vi "Control Panel Controller.vi"(8 "error in":errorcluster) -> ()   [LabVIEW 2019]
doc: "This VI executes continuously carrying out the current operation and responding to updates or new operations. It will often contain the timing or control code that is difficult to place directly in TeleOp. This VI generally opens all sensors and motors and isolates the rest of the robot code from knowing how the operations are carried out."
uses:
  <vilib>/Rock Robotics/WPI/Framework/Completion Status.ctl
  Control Panel Setpoints.ctl
  Control Panel Operations.ctl
  <vilib>/Rock Robotics/WPI/ThirdParty/Phoenix-LabVIEW/Motor Controller/Controls/CTRE_Phoenix_MotorControl_ControlMode.ctl
  Framework/Robot Global Data.vi
  <vilib>/Rock Robotics/Network Tables/NT Write Number.vi
panel:
  in  "Interactive Values":T1
  out "Current\nCmd":string
  in  "Buttons":cluster{"Execute Cmd":bool, "Abort Cmd":bool}
  out "Command Timing":cluster{"Start Time (ms)":u32, "Iterations":i32}
  out "Status":T3
  # "Tip: It may be helpful to observe inputs and sensor values.\nYou may also want to display tuning or debugging controls."
  # "Interactive Command: You may fill in the settings for a command\nand schedule it with the Execute button. You can observe and abort\nany command while fine tuning the code for the controller."
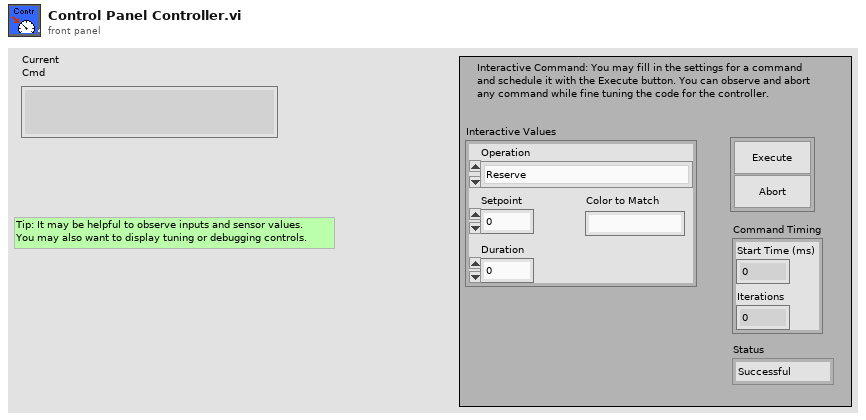
[diagram p1: front panel]
types:
  T1 = typedef "Control Panel Setpoints.ctl" = cluster{"Operation":T2, "Setpoint":dbl, "Duration":dbl, "Color to Match":string}
  T2 = typedef "Control Panel Operations.ctl" = enum16{"Reserve", "Read Current", "Immediate", "Move for Time", "Three Turns", "Match Color"}
  T3 = typedef "Completion Status.ctl" = enum16{"Successful", "Aborted", "Incomplete"}
  T4 = typedef "WPI_MotorControlDeviceRef.ctl" = cluster{"DeviceStatus":errorcluster, "Type":T5, "PWM":cluster{"PWM Channel":T6, "DeadBand":T7}, "CAN":cluster{"Device Number":u8, "SetOutput VI Ref":variant, "GetOutput VI Ref":variant, "Enable VI Ref":variant, "Disable VI Ref":variant, "Data":variant}, "Invert":bool, "DIO PWM":cluster{"PWM \"Enable\" Channel":T6, "DIOChannel":T8, "PWM Rate":dbl}}
  T5 = typedef "WPI_MotorControlType.ctl" = enum16{"PWM", "CAN", "DIO PWM"}
  T6 = typedef "FPGA_DIOPWMChannel.ctl" = enum8{"PWM 0", "PWM 1", "PWM 2", "PWM 3", "PWM 4", "PWM 5", "PWM 6", "PWM 7", "PWM 8", "PWM 9", "PWM MXP 0", "PWM MXP 1", "PWM MXP 2", "PWM MXP 3", "PWM MXP 4", "PWM MXP 5", "PWM MXP 6", "PWM MXP 7", "PWM MXP 8", "PWM MXP 9", "Invalid"}
  T7 = typedef "WPI_PWMDeadband.ctl" = cluster{"Name":string, "maxPositivePwm":i32, "minPositivePwm":i32, "centerPwm":i32, "maxNegativePwm":i32, "minNegativePwm":i32, "angularRange":u16}
  T8 = typedef "FPGA_DIOChannel.ctl" = enum8{"DIO 0", "DIO 1", "DIO 2", "DIO 3", "DIO 4", "DIO 5", "DIO 6", "DIO 7", "DIO 8", "DIO 9", "DIO MXP 0", "DIO MXP 1", "DIO MXP 2", "DIO MXP 3", "DIO MXP 4", "DIO MXP 5", "DIO MXP 6", "DIO MXP 7", "DIO MXP 8", "DIO MXP 9", "DIO MXP 10", "DIO MXP 11", "DIO MXP 12", "DIO MXP 13", "DIO MXP 14", "DIO MXP 15", "SPI Port CS1", "SPI Port CS2", "SPI Port CS3", "SPI Port MISO", "SPI Port MOSI", "Invalid"}
  T9 = typedef "Command Status Info.ctl" = cluster{"Name":string, "Status":T3, "notifier out":T10}
  T10 = typedef "Completion Notifier.ctl" = refnum<notifier>
  T11 = cluster{"Current Command":T1, "Command Timing":cluster{"Start Time (ms)":u32, "Iterations":i32}, "Command Arguments":cluster{"Command Info":T9, "Description":string, "Default Command":T1, "queue out":refnum<queue>, "Subsystem Name":string}}
  T12 = typedef "CTRE_Phoenix_MotorControl_ControlMode.ctl" = u16
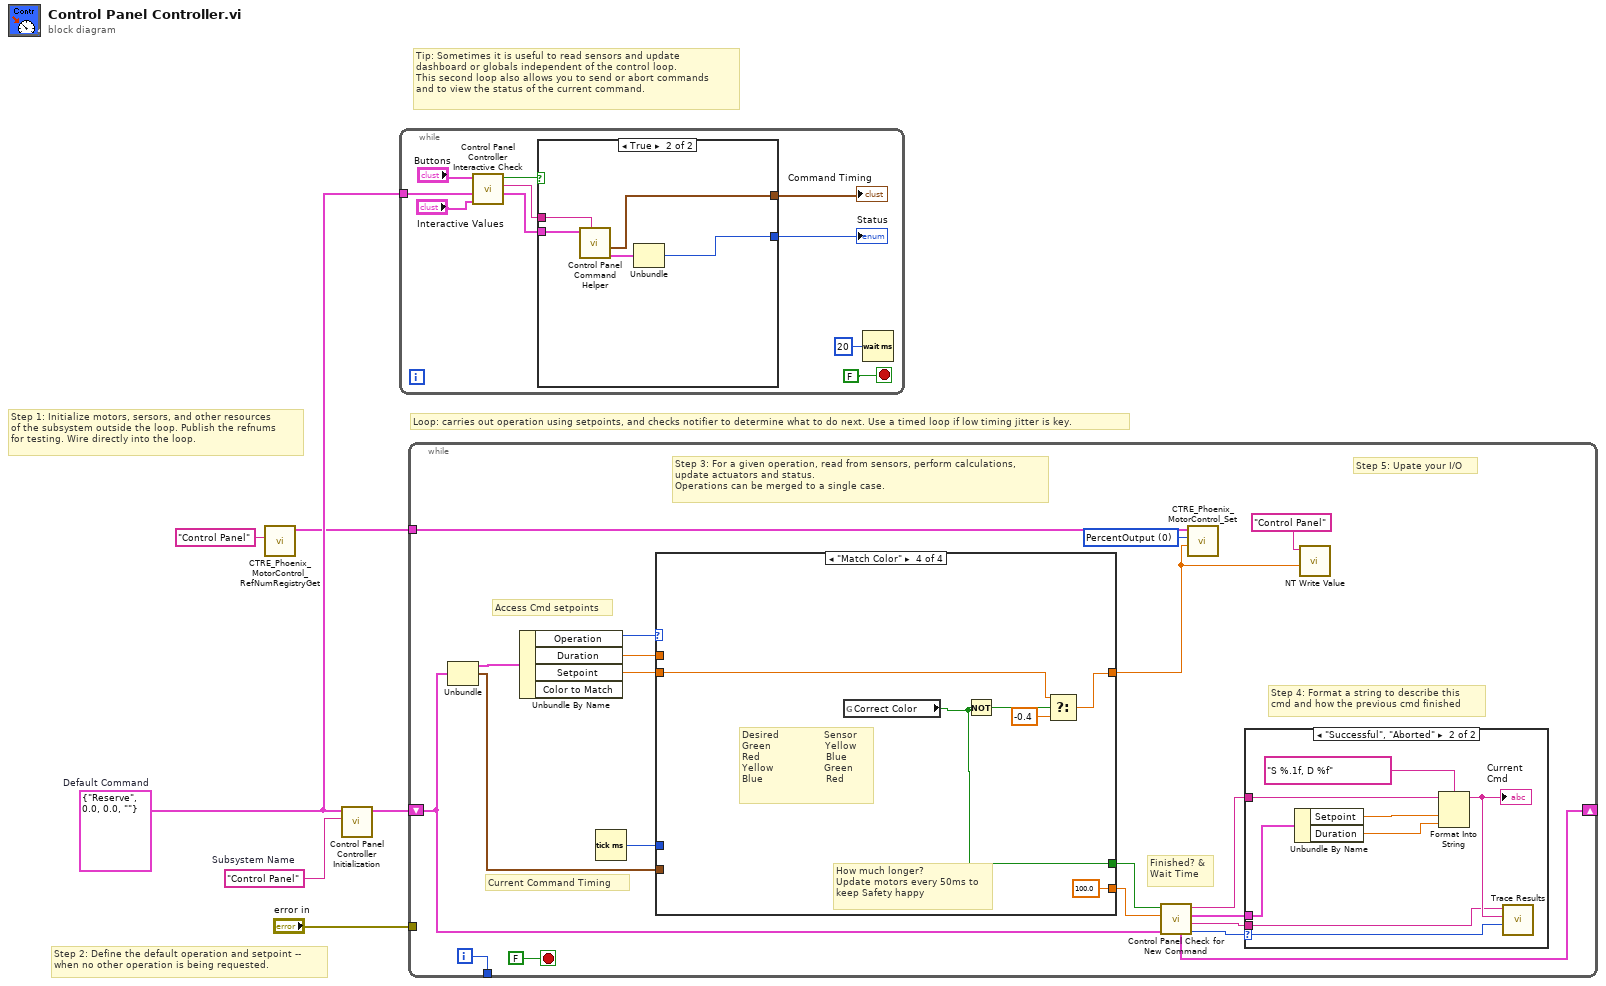
[diagram p0: block diagram]
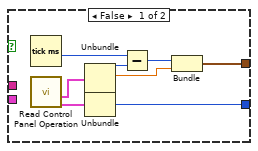
[diagram p2: hidden frame]
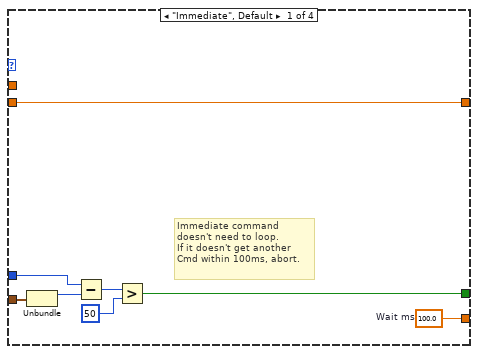
[diagram p4: hidden frame]
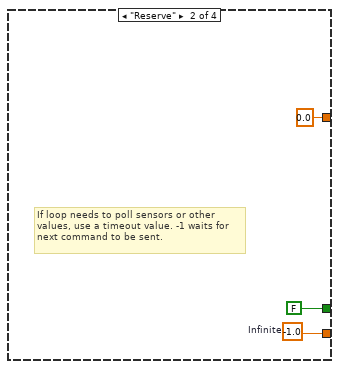
[diagram p5: hidden frame]
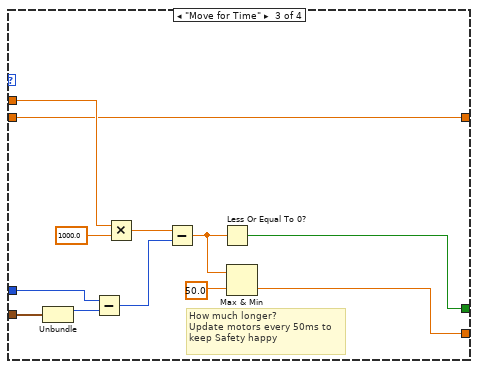
[diagram p6: hidden frame]
diagram:
  w3 = T1 {"Operation"=enum."Reserve", "Setpoint"=0.0, "Duration"=0.0, "Color to Match"=""}  # Default Command
  w4 = "Control Panel"  # Subsystem Name
  # "Tip: Sometimes it is useful to read sensors and update\ndashboard or globals independent of the control loop.\nThis second loop also allows you to send or abort commands\nand to view the status of the current command."
  # "Step 2: Define the default operation and setpoint --\nwhen no other operation is being requested."
  # "Step 1: Initialize motors, sersors, and other resources\nof the subsystem outside the loop. Publish the refnums\nfor testing. Wire directly into the loop."
  # "Loop: carries out operation using setpoints, and checks notifier to determine what to do next. Use a timed loop if low timing jitter is key."
  n1 = call <vilib>:"CTRE_Phoenix_MotorControl_RefNumRegistryGet.vi"("refnum name"="Control Panel") -> ("PhoenixMotorControlDevRef"=w1:T4)  [unwired: 9 in, 1 out]
  n2 = call "Control Panel Controller Initialization.vi"("Subsystem Name"=w4, "Default Command"=w3) -> ("Current Command"=w5:T11)  [unwired: 9 in]
  n3 = while {
    tunnel: w3 -> [w13]
    stop <- FALSE stop-if-true
    n4 = call "Control Panel Controller Interactive Check.vi"("Interactive Command in"="Interactive Values", "Default Command"=w13, "Buttons"="Buttons") -> ("Interactive Command out"=w10:T1, "Trace String"=w11:string, "Schedule"=w12:bool)  [unwired: 6 in]
    n5 = case shown="True" w12 {
      tunnel: [w24 w29] -> w9
      tunnel: w10 -> [_ w27]
      tunnel: [w20 w25] -> w8
      tunnel: w11 -> [_ w28]
      frame False {
        n6 = Tick Count (ms)() -> (millisecond timer value=w19:u32)
        n7 = call "Read Control Panel Operation.vi"() -> ("Command Info"=w17:T9, "SubSystem Data"=w18:T1)  [unwired: 9 in, 1 out]
        n8 = Unbundle(w18) -> ("Operation"=w23:T2, "Setpoint"=w21:dbl)  [unwired: 2 out]
        n9 = Unbundle(w17) -> ("Status"=w24:T3)  [unwired: 2 out]
        n10 = Subtract(x=w19, y=w23) -> (x-y=w22:u32)
        n11 = Bundle(w22, "Setpoint"=w21) -> (w20:cluster{u32, "Setpoint":dbl})  [unwired: 1 in]
      }
      frame True {
        n12 = call "Control Panel Command Helper.vi"("Description"=w28, "SubSystem Data"=w27) -> ("Command Info Out"=w26:T9, "Command Timing"=w25:cluster{"Start Time (ms)":u32, "Iterations":i32})  [unwired: 7 in, 1 out]
        n13 = Unbundle(w26) -> ("Status"=w29:T3)  [unwired: 2 out]
      }
    }
    "Status" <- w9
    "Command Timing" <- w8
    n14 = Wait (ms)(milliseconds to wait=u32 20) -> ()  [unwired: 1 out]
  }
  n15 = while {
    shift-right: [w41] -> _
    shift-left: w5 -> [w34]
    tunnel: [w48] -> _
    tunnel: "error in" -> [_]
    tunnel: w1 -> [w33]
    i -> [w48]
    stop <- FALSE stop-if-true
    w32 = T12 0 items=["PercentOutput"=0, "Position"=1, "Velocity"=2, "Current"=3, "Follower"=5, "MotionProfile"=6, "MotionMagic"=7, "MotionProfileArc"=10, "Disabled"=15] ("Control Mode")
    # "Step 5: Upate your I/O"
    # "Step 4: Format a string to describe this\ncmd and how the previous cmd finished"
    # "Current Command Timing"
    # "Access Cmd setpoints"
    # "Finished? &\nWait Time"
    # "Step 3: For a given operation, read from sensors, perform calculations,\nupdate actuators and status.\nOperations can be merged to a single case."
    n16 = Unbundle(w34) -> ("Current Command"=w47:T1, "Command Timing"=w43:cluster{"Start Time (ms)":u32, "Iterations":i32})  [unwired: 1 out]
    n17 = Unbundle By Name(w47) -> ("Operation"=w46:T2, "Duration"=w45:dbl, "Setpoint"=w42:dbl)  [unwired: 1 out]
    n18 = Tick Count (ms)() -> (millisecond timer value=w44:u32)
    n19 = case shown="\"Match Color\"" w46 {
      tunnel: [w65 w68 w72 100.0 ("Infinite")] -> w39
      tunnel: [w59 FALSE ("ignore previous (F)") w71 w81] -> w40
      tunnel: w43 -> [w61 _ w73 _]
      tunnel: w45 -> [_ _ w70 _]
      tunnel: w44 -> [w60 _ w74 _]
      tunnel: w42 -> [w58 _ w69 w83]
      tunnel: [w58 0.0 ("Setpoint") w69 w82] -> w30
      frame "Immediate", Default {
        w65 = 100.0  # Wait ms
        # "Immediate command\ndoesn't need to loop.\nIf it doesn't get another\nCmd within 100ms, abort."
        n20 = Unbundle(w61) -> ("Start Time (ms)"=w64:u32)  [unwired: 1 out]
        n21 = Subtract(x=w60, y=w64) -> (x-y=w63:u32)
        n22 = Greater?(x=w63, y=u8 50 ("Left Motor")) -> (0:w59:bool)
      }
      frame "Reserve" {
        w68 = -1.0  # Infinite
        # "If loop needs to poll sensors or other\nvalues, use a timeout value. -1 waits for\nnext command to be sent."
      }
      frame "Move for Time" {
        # "How much longer?\nUpdate motors every 50ms to\nkeep Safety happy"
        n23 = Unbundle(w73) -> ("Start Time (ms)"=w77:u32)  [unwired: 1 out]
        n24 = Subtract(x=w74, y=w77) -> (x-y=w80:u32)
        n25 = Multiply(x=w70, y=1000.0) -> (x*y=w79:dbl)
        n26 = Subtract(x=w79, y=w80) -> (x-y=w76:dbl)
        n27 = Less Or Equal To 0?(x=w76) -> (x <= 0?=w71:bool)
        n28 = Max & Min(x=w76, y=50.0) -> (min(x,y)=w72:dbl)  [unwired: 1 out]
      }
      frame "Match Color" {
        # "Desired               Sensor\nGreen                  Yellow\nRed                      Blue       \nYellow                 Green\nBlue                     Red"
        # "How much longer?\nUpdate motors every 50ms to\nkeep Safety happy"
        n29 = global read "Robot Global Data.vi" "Correct Color"() -> (w81:bool)
        n30 = Not(x=w81) -> (.not. x?=w85:bool)
        n31 = Select(t=w83, s=w85, f=-0.4) -> (s? t:f=w82:dbl)
      }
    }
    n32 = call "Control Panel Check for New Command.vi"("Current Command"=w34, "Wait time (ms)"=w39, "Finished?"=w40) -> ("Completion"=w35:T3, "Subsystem Name"=w36:string, "Current Command"=w37:T1, "Initial Trace String"=w38:string, "NextCommand"=w41:T11)  [unwired: 4 in]
    n33 = call <vilib>:"CTRE_Phoenix_MotorControl_Set.vi"("Output"=w30, "Control Mode"=w32, "PhoenixMotorControlDevRef"=w33) -> ()  [unwired: 7 in, 2 out]
    n34 = case shown="\"Successful\", \"Aborted\"" w35 {
      selector: w35 -> [_ w57]
      tunnel: w38 -> [_ w53]
      tunnel: w37 -> [_ w54]
      tunnel: w36 -> [_ w50]
      frame "Incomplete", Default {
        # "Continuing current command"
      }
      frame "Successful", "Aborted" {
        # "Report and setup for next command"
        n35 = Unbundle By Name(w54) -> ("Setpoint"=w56:dbl, "Duration"=w51:dbl)
        n36 = Format Into String(format string="S %.1f, D %f", initial string=w53, w56, w51) -> (resulting string=w52:string)  [unwired: 1 in, 1 out]
        "Current\nCmd" <- w52
        n37 = call <vilib>:"Trace Results.vi"("Status of previous command"=w57, "Description"=w52, "Subsystem"=w50) -> ()  [unwired: 9 in]
      }
    }
    n38 = call-poly <vilib>:"NT Write Value.vi"("Numeric"=w30, "Name"="Control Panel" ("refnum name")) -> ()  [unwired: 9 in, 1 out]
  }
